vi "VCS Get Controller Gain.vi"(8 "error in (no error)":errorcluster, 10 "controller gain":cluster{"controller":u16, "gain":u16}={"controller"=1, "gain"=1} {"gain" items=["P-Gain"=1, "I-Gain"=2, "D-Gain"=3, "Feedforward Velocity Gain"=10, "Feedforward Acceleration Gain"=11, "Theta Gain"=20, "Omega Gain"=21, "Tau Gain"=22, "P Gain low"=101, "P Gain high"=102, "Gain Scheduling Weight"=110, "Filter Coefficient A"=120, "Filter Coefficient B"=121, "Filter Coefficient C"=122, "Filter Coefficient D"=123, "Filter Coefficient E"=124]; "controller" items=["PI Current Controller"=1, "PI Velocity Controller"=10, "PI Velocity Controller with Observer"=11, "PID Position Controller"=20, "Dual Loop Position Controller"=21]}, 11 "axis in":cluster{"keyHandle":u32, "nodeId":u16}={"keyHandle"=0, "nodeId"=1}) -> (0 "error out":errorcluster, 2 "value":u64, 3 "axis out":cluster{"keyHandle":u32, "nodeId":u16}={"keyHandle"=0, "nodeId"=1})   [LabVIEW 2017, in "maxonEPOS.lvlib"]
doc: "<B>VCS Get Current Regulator Gain</B> reads all current regulator gains."
uses:
  Examples/maxonEPOS.lvlib
  SSI_Tool/InstrumentsInterfaces/Motordriver/maxon EPOS/Resources/EposCmd64.dll
  SSI_Tool/InstrumentsInterfaces/Motordriver/maxon EPOS/Resources/EposCmd.dll
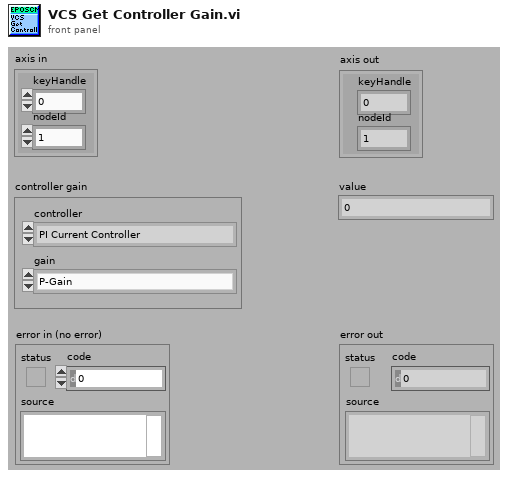
[diagram p1: front panel]
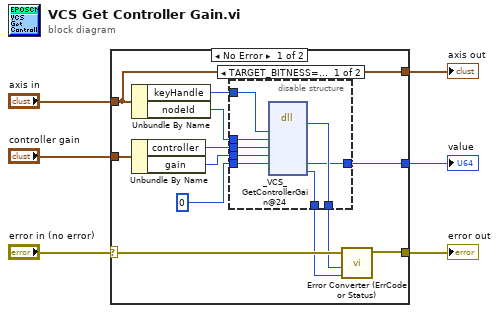
[diagram p0: block diagram]
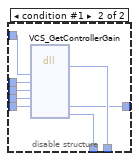
[diagram p2: hidden frame]
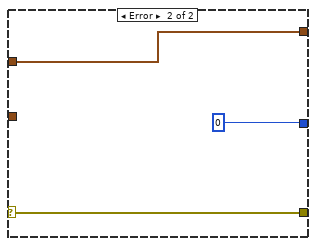
[diagram p3: hidden frame]
diagram:
  n1 = case shown="No Error" "error in (no error)" {
    selector: "error in (no error)" -> [w18 w37]
    tunnel: [w17 w37] -> w5
    tunnel: "axis in" -> [w13 w36]
    tunnel: [w13 w36] -> w3
    tunnel: [w11 u64 0 ("pI")] -> w2
    tunnel: "controller gain" -> [w9 _]
    frame No Error {
      n2 = Unbundle By Name(w13) -> ("keyHandle"=w15:u32, "nodeId"=w14:u16)
      n3 = Unbundle By Name(w9) -> ("controller"=w8:u16, "gain"=w7:u16)
      n4 = disable-structure shown="TARGET_BITNESS==32, Standard" {
        disable-tunnel: [w26 w34] -> w16
        disable-tunnel: w15 -> [w25 w33]
        disable-tunnel: w14 -> [w24 w32]
        disable-tunnel: [w23 w31] -> w12
        disable-tunnel: [w22 w27] -> w11
        disable-tunnel: u64 0 ("pErrorCode") -> [w21 w30]
        disable-tunnel: w8 -> [w20 w29]
        disable-tunnel: w7 -> [w19 w28]
        frame condition #0 (active) {
          n5 = dll-call lib="C:/workspace/project/scancon/sw/SSI_Tool/InstrumentsInterfaces/Motordriver/maxon EPOS/Resources/EposCmd.*" fn="_VCS_GetControllerGain@24" ("EposCmd.dll:_VCS_GetCurrentRegulatorGain@20")("KeyHandle"=w25, "NodeId"=w24, "Controller"=w20, "Gain"=w19, "pValue"=w21) -> ("Rückgabetyp"=w23:i32, "pValue"=w22:u64, "pErrorCode"=w26:u32)  [unwired: 8 in, 2 out]
        }
        frame condition #1 {
          n6 = dll-call lib="C:/Sources/LabView/maxon EPOS/Resources/EposCmd64.dll" fn="VCS_GetControllerGain" ("EposCmd.dll:_VCS_GetCurrentRegulatorGain@20")("KeyHandle"=w33, "NodeId"=w32, "Controller"=w29, "Gain"=w28, "pValue"=w30) -> ("Rückgabetyp"=w31:i32, "pValue"=w27:u64, "pErrorCode"=w34:u32)  [unwired: 8 in, 2 out]
        }
      }
      n7 = call "Error Converter (ErrCode or Status).vi"("error code"=w16, "return type"=w12, "error in (no error)"=w18) -> ("error out"=w17:errorcluster)  [unwired: 7 in]
    }
    frame Error {
    }
  }
  "error out" <- w5
  "axis out" <- w3
  "value" <- w2
